vi "系统设置全局变量.vi"() -> ()   [LabVIEW 2016]
panel:
  in  "系统重启设置":T1 {"分" max=59 format="%02.0f"; "时" max=23 format="%02.0f"}
  in  "首页显示信息设置":T2={"水温"=FALSE, "pH"=FALSE, "DO"=FALSE, "Cond"=FALSE, "Turb"=FALSE, "氨氮"=FALSE, "总磷"=FALSE, "总氮"=FALSE, "CODMn"=FALSE, "CODCr"=FALSE, "水位"=FALSE, "流速"=FALSE, "瞬时流量"=FALSE, "室温"=TRUE, "湿度"=TRUE}
  in  "流量阈值":dbl=4.0 min=1.0 max=24.0
  in  "时间阈值":u16=4 min=1 max=24
  in  "超标留样启用":bool caption="采配水禁用"
  in  "周期设置":enum16{"自由设定", "国标协议", "流量设定"}(ring)
  in  "运行间隔":i16=4 min=1 max=24
  in  "跨度核查时间":u16(ring)=6 items=["00H", "01H", "02H", "03H", "04H", "05H", "06H", "07H", "08H", "09H", "10H", "11H", "12H", "13H", "14H", "15H", "16H", "17H", "18H", "19H", "20H", "21H", "22H", "23H"]
  in  "空白核查时间":u16(ring)=2 items=["00H", "01H", "02H", "03H", "04H", "05H", "06H", "07H", "08H", "09H", "10H", "11H", "12H", "13H", "14H", "15H", "16H", "17H", "18H", "19H", "20H", "21H", "22H", "23H"]
  in  "质控启动日期":string(combo)="关闭"
  in  "CODCr自动启动设置":bool
  in  "总磷总氮自动启动设置":bool
  in  "氨氮自动启动设置":bool
  in  "CODmn自动启动设置":bool
  in  "多参数自动启动设置":bool
  in  "运行模式":enum16{"维护模式", "常规模式", "应急模式", "质控模式"}(ring)
  in  "24H周期设置":bool[](xcontrol)
  in  "多参数启用":bool caption="多参数禁用"
  in  "其他启用":bool caption="其他禁用"
  in  "电源管理启用":bool caption="电源管理禁用"
  in  "流量计启用":bool caption="流量计禁用"
  in  "质控单元启用":bool caption="质控单元禁用"
  in  "总磷总氮启用":bool caption="总磷总氮禁用"
  in  "氨氮启用":bool caption="氨氮禁用"
  in  "CODcr启用":bool caption="CODcr禁用"
  in  "CODMn启用":bool caption="CODMn禁用"
  in  "采配水启用":bool caption="采配水禁用"
  # "质控频次："
  # "空白核查时间："
  # "跨度核查时间："
  # "频次："
  # "时间："
  # "："
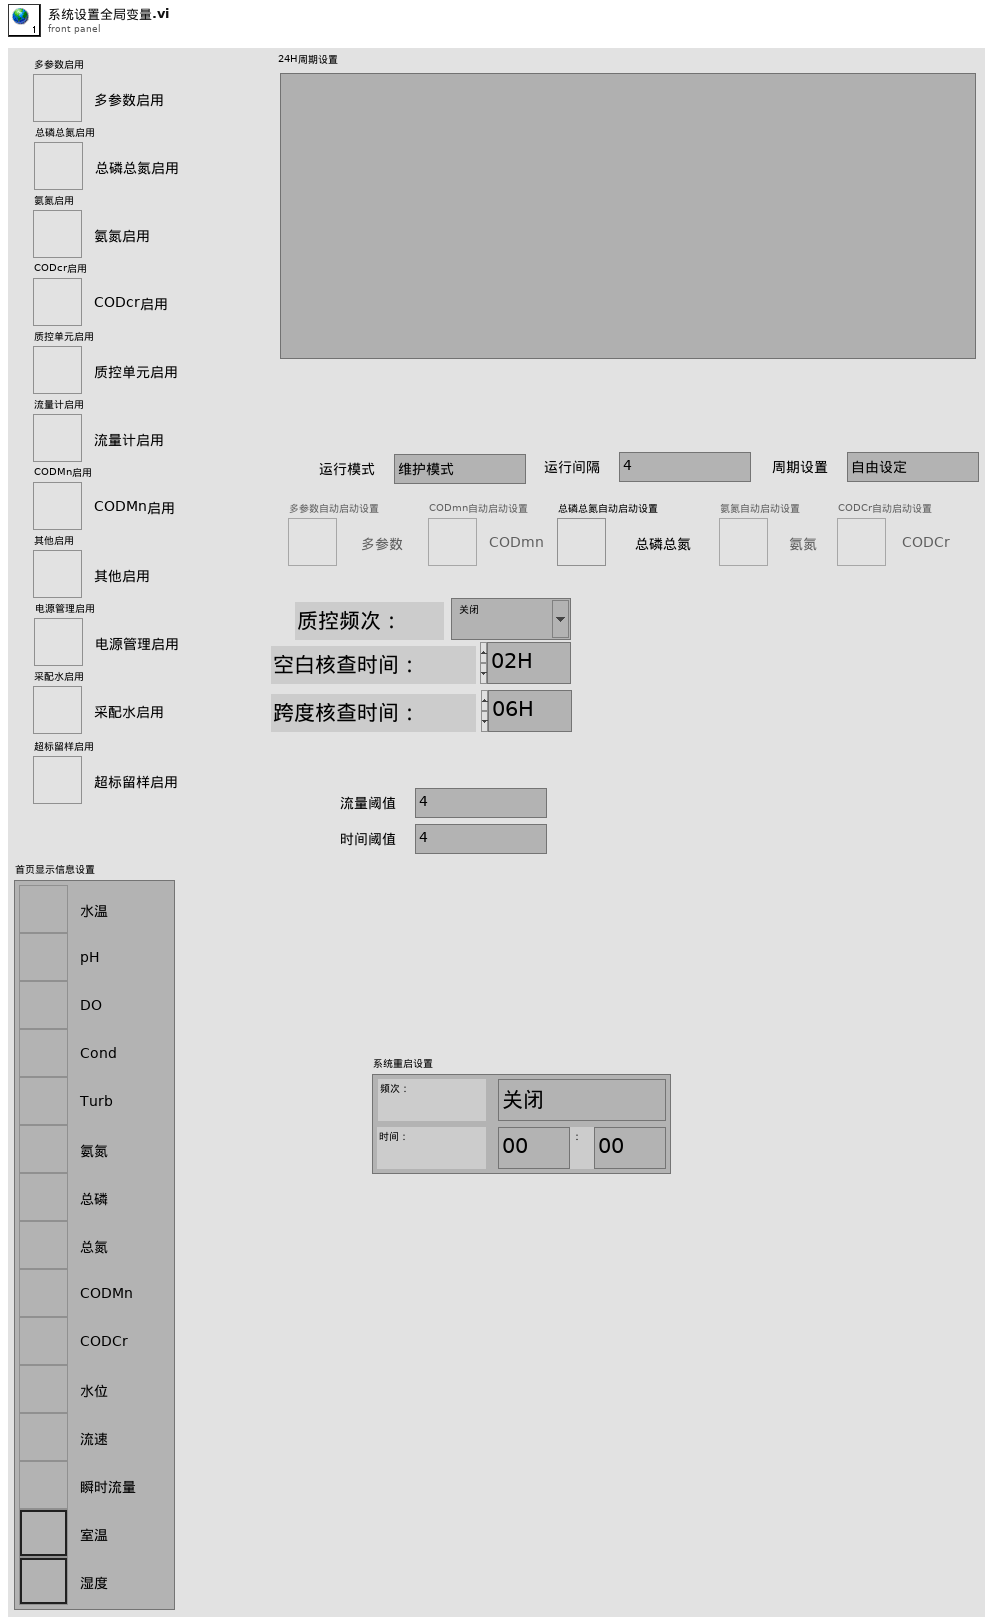
[diagram p1: front panel]
types:
  T1 = cluster{"频次":enum16{"关闭", "每天", "星期一", "星期二", "星期三", "星期四", "星期五", "星期六", "星期日"}, "时":u16, "分":u16}
  T2 = cluster{"水温":bool, "pH":bool, "DO":bool, "Cond":bool, "Turb":bool, "氨氮":bool, "总磷":bool, "总氮":bool, "CODMn":bool, "CODCr":bool, "水位":bool, "流速":bool, "瞬时流量":bool, "室温":bool, "湿度":bool}
diagram:
